vi "Create All Message Queues.vi"(8 "error in (no error)":errorcluster) -> (0 "error out":errorcluster, 3 "Message Queues out":T1)   [LabVIEW 2018, in "Message Queue.lvlib"]
doc: "This VI creates and initializes all the message queues for your application. If your application requires more than one message queue, right-click the \"Message Queues\" constant above and select Open Type Def. Add the new Message Queue(s) to the type definition, then initialize them in this VI."
uses:
  Message Queue.lvlib
  All Message Queues.ctl
  Message Cluster.ctl
  Enqueue Message (Single).vi
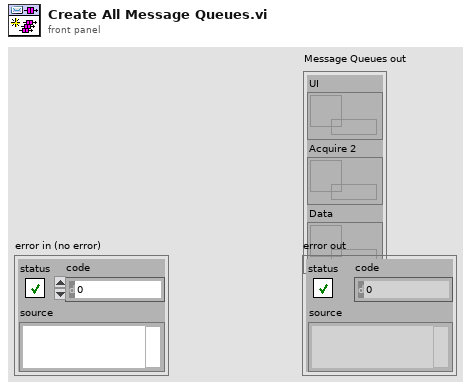
[diagram p1: front panel]
types:
  T1 = typedef "Message Queue.lvlib/All Message Queues.ctl" = cluster{"UI":refnum<queue>, "Acquire 2":refnum<queue>, "Data":refnum<queue>}
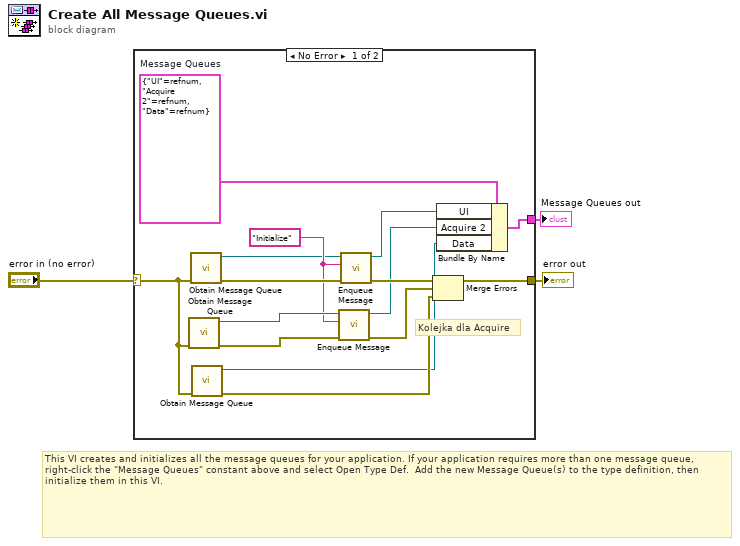
[diagram p0: block diagram]
diagram:
  # "This VI creates and initializes all the message queues for your application. If your application requires more than one message queue, right-click the \"Message Queues\" constant above and select Open Type Def.  Add the new Message Queue(s) to the type definition, then initialize them in this VI."
  n1 = case shown="No Error" "error in (no error)" {
    selector: "error in (no error)" -> [w6 w19]
    tunnel: [w8 w19] -> w3
    tunnel: [w16 _] -> w2
    frame No Error {
      w12 = "Initialize" ("Message")
      w17 = T1 {"UI"=refnum, "Acquire 2"=refnum, "Data"=refnum}  # Message Queues
      # "Kolejka dla Acquire"
      n2 = call "Obtain Message Queue.vi"("error in (no error)"=w6) -> ("error out"=w14:errorcluster, "Message Queue"=w13:refnum<queue>)  [unwired: 9 in]
      n3 = call "Obtain Message Queue.vi"("error in (no error)"=w6) -> ("error out"=w15:errorcluster, "Message Queue"=w11:refnum<queue>)  [unwired: 9 in]
      n4 = call "Obtain Message Queue.vi"("error in (no error)"=w6) -> ("error out"=w5:errorcluster, "Message Queue"=w4:refnum<queue>)  [unwired: 9 in]
      n5 = call-poly "Enqueue Message.vi"("error in (no error)"=w14, "Message"=w12, "Message Queue"=w13) -> ("error out"=w7:errorcluster, "dup Message Queue"=w9:refnum<queue>)  [unwired: 7 in]
      n6 = call-poly "Enqueue Message.vi"("error in (no error)"=w15, "Message"=w12, "Message Queue"=w11) -> ("error out"=w18:errorcluster, "dup Message Queue"=w10:refnum<queue>)  [unwired: 7 in]
      n7 = Merge Errors(w18, w7, w5) -> (w8:errorcluster)
      n8 = Bundle By Name(cluster=w17, "UI"=w10, "Acquire 2"=w9, "Data"=w4) -> (w16:T1)
    }
    frame Error {
    }
  }
  "Message Queues out" <- w2
  "error out" <- w3
